vi "PH_Names.Famous Tagnames.vi"() -> (0 "Laser Enabling.DIM Service Name":string, 1 "PreAmp Enabling.DIM Service Name":string, 4 "Timing Mode.DIM Service Name":string, 5 "MainAmp Enabling.DIM Service Name":string, 6 "Enabling Exp. 1.DIM Service Name":string, 7 "Enabling Exp. 2.DIM Service Name":string, 8 "Emergency Off.DIM Service Name":string, 9 "Enabling Exp. 3.DIM Service Name":string, 10 "Enabling Exp. 4.DIM Service Name":string)   [LabVIEW 2014, in "PH_Common.lvlib"]
uses:
  PH_Common.lvlib
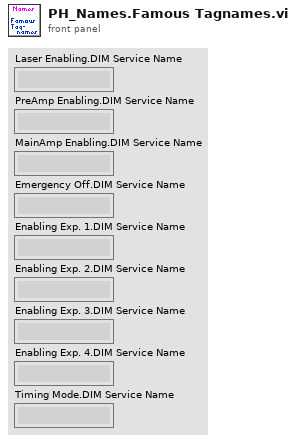
[diagram p1: front panel]
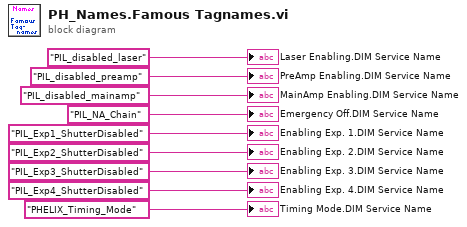
[diagram p0: block diagram]
diagram:
  "Timing Mode.DIM Service Name" <- "PHELIX_Timing_Mode" ("Timing Mode.DIM Service Name")
  "Enabling Exp. 4.DIM Service Name" <- "PIL_Exp4_ShutterDisabled" ("Enabling Exp. 4.DIM Service Name")
  "Enabling Exp. 3.DIM Service Name" <- "PIL_Exp3_ShutterDisabled" ("Enabling Exp. 3.DIM Service Name")
  "Enabling Exp. 2.DIM Service Name" <- "PIL_Exp2_ShutterDisabled" ("Enabling Exp. 2.DIM Service Name")
  "Enabling Exp. 1.DIM Service Name" <- "PIL_Exp1_ShutterDisabled" ("Enabling Exp. 1.DIM Service Name")
  "Emergency Off.DIM Service Name" <- "PIL_NA_Chain" ("Emergency Off.DIM Service Name")
  "MainAmp Enabling.DIM Service Name" <- "PIL_disabled_mainamp" ("MainAmp Enabling.DIM Service Name")
  "PreAmp Enabling.DIM Service Name" <- "PIL_disabled_preamp" ("PreAmp Enabling.DIM Service Name")
  "Laser Enabling.DIM Service Name" <- "PIL_disabled_laser" ("Laser Enabling.DIM Service Name")
